vi "AWContainerWrite.vi"(1 "Input":i16[](array[numeric])=[0]) -> ()   [LabVIEW 2010, in "Recorder.lvlib"]
uses:
  Recorder.lvlib
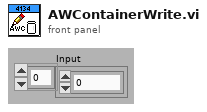
[diagram p1: front panel]
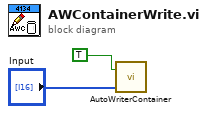
[diagram p0: block diagram]
diagram:
  n1 = call "AutoWriterContainer.vi"("Mode(Write=True)"=TRUE, "Input"="Input") -> ()  [unwired: 1 out]
